vi "CIETallnodesReactor.vi"() -> ()   [LabVIEW 2017]
uses:
  <vilib>/OPCUA/controls/Write Status.ctl
  <vilib>/OPCUA/controls/NodeId.ctl
  <vilib>/OPCUA/controls/Subscription Data Change.ctl
  <vilib>/OPCUA/controls/Data Type.ctl
  <vilib>/OPCUA/controls/OPC UA StatusCode.ctl
  <vilib>/OPCUA/controls/Subscription ID.ctl
  <vilib>/OPCUA/controls/OPC UA Client Refnum.ctl
  <vilib>/OPCUA/controls/NodeIds.ctl
  <vilib>/OPCUA/client/Multiple Write Bool.vi
  <vilib>/OPCUA/client/Multiple Write Double.vi
  <vilib>/OPCUA/NI OPC UA Client.lvlib
panel:
  out "CX-114":dbl format="%.1f"
  out "CX-113":dbl format="%.1f"
  out "CX-112":dbl format="%.1f"
  out "CX-111":dbl format="%.1f"
  out "CX-104":dbl format="%.1f"
  out "CX-103":dbl format="%.1f"
  out "CX-102":dbl format="%.1f"
  out "CX-101":dbl format="%.1f"
  out "ST-14w":dbl format="%.1f"
  out "ST-14s":dbl format="%.1f"
  out "ST-14n":dbl format="%.1f"
  out "ST-14e":dbl format="%.1f"
  out "ST-12sw":dbl format="%.1f"
  out "ST-12se":dbl format="%.1f"
  out "ST-12n":dbl format="%.1f"
  in  "Flow Data?":bool=TRUE
  in  "CTAH Set Point":sgl format="%.1f"
  in  "Mode":string(combo)
  out "Server OK":bool
  out "System Time [s]":dbl
  out "Power Output":dbl(graph)
  out "Frequency [Hz] 3":dbl(slide) scale=0.0..60.0
  out "Frequency [Hz] 2":dbl(slide) scale=0.0..60.0
  out "Frequency [Hz]":dbl(knob) scale=0.0..45.0
  out "Power [W]":dbl(slide) caption="Power Output [W]" scale=0.0..10000.0
  in  "Desired Power [W]":dbl min=0.0 max=10000.0 step=1.0 format="%.1f"
  out "WT-10":dbl format="%.1f"
  out "BT-11":dbl format="%.1f"
  out "BT-12":dbl format="%.1f"
  out "WT-13":dbl format="%.1f"
  out "WT-20":dbl format="%.1f"
  out "BT-21":dbl format="%.1f"
  out "WT-22":dbl format="%.1f"
  out "BT-23":dbl format="%.1f"
  out "WT-24":dbl format="%.1f"
  out "BT-25":dbl format="%.1f"
  out "WT-26":dbl format="%.1f"
  out "BT-27":dbl format="%.1f"
  out "WT-28":dbl format="%.1f"
  out "BT-29":sgl format="%.1f"
  out "BT-30":dbl format="%.1f"
  out "WT-31":dbl format="%.1f"
  out "BT-32":dbl format="%.1f"
  out "WT-33":dbl format="%.1f"
  out "BT-34":dbl format="%.1f"
  out "WT-35":dbl format="%.1f"
  out "WT-40":dbl format="%.1f"
  out "BT-41":dbl format="%.1f"
  out "WT-42":dbl format="%.1f"
  out "BT-43":dbl format="%.1f"
  out "BT-60":dbl format="%.1f"
  out "WT-61":dbl format="%.1f"
  out "WT-62":dbl format="%.1f"
  out "BT-63":dbl format="%.1f"
  out "WT-64":dbl format="%.1f"
  out "BT-65":sgl format="%.1f"
  out "BT-66":dbl format="%.1f"
  out "WT-67":dbl format="%.1f"
  out "ST-10":dbl format="%.1f"
  out "ST-11":dbl format="%.1f"
  out "ST-13":dbl format="%.1f"
  out "AT-01":dbl format="%.1f"
  out "AT-02":dbl format="%.1f"
  in  "Power Output On":bool
  in  "ACTIVATE - CTAH":bool
  in  "ACTIVATE - TCHX":bool
  in  "TCHX Frequency [Hz]":sgl min=0 max=60 step=0.1 format="%.1f"
  in  "ACTIVATE - PUMP":bool
  in  "Pump Frequency [Hz]":dbl min=0.0 max=45.0 step=0.10000000149011612 format="%.1f"
  out "DHX Primary Flow\n\n\nFM-20 [kg/s]":dbl format="%.3f"
  out "Bypass Flow\n\n\nFM-30 [kg/s]":dbl format="%.3f"
  out "Primary Flow\n\n\nFM-40 [kg/s]":dbl format="%.3f"
  out "DRACS Flow\n\n\nFM-60 [kg/s]":dbl format="%.3f"
  out "System Safe":bool
  in  "Exit Profile":bool
  in  "Select Operation Mode":T1(ring) caption="Select Operation Mode2"
  in  "Load Power Profile":bool
  in  "Dyn. Power Profile File":path
  out "CTAH Temperatures":cluster{"CTAH Outlet":dbl, "CTAH Inlet":dbl}(graph)
  out "Core Temperatures":cluster{"Heater Inlet":dbl, "Heater Outlet":dbl}(graph)
  out "Profile Step":i32
  in  "Stop Reactor Interface":bool
  in  "error in (no error)":errorcluster
  out "Connection Status":bool
  in  "Stop":bool
  in  "Disconnect":bool
  in  "Connect to Server":bool
  out "activateTchx":bool
  out "activatePump":bool
  out "activateCtah":bool
  out "20001":dbl
  out "operatorActions":string
  out "chat":string
  out "spoofEnabled":bool
  out "flowData":dbl
  out "exitProfile":bool
  out "actionRecorderOn":bool
  out "powerOutputOn":bool
  out "powerInputSignal":dbl
  out "outputVoltage2":dbl
  out "outputVoltage1":dbl
  out "outputCurrent2":dbl
  out "outputCurrent1":dbl
  out "tchxTempInResGen":dbl
  out "matlabActive":bool
  out "heaterTempOutResGen":dbl
  out "heaterResGen":dbl
  out "faultDiagnosticsActive":bool
  out "dhxTempOutResGen":dbl
  out "ctahTempInResGen":dbl
  out "CTAHResGen":bool
  out "Temperature":dbl
  out "Message":string
  out "Sensor Status":bool
  out "Time Stamp 2":timestamp
  # "DRACS"
  # "PRIMARY"
  # "HOT DRACS"
  # "DHX TOP"
  # "TCHX"
  # "HOT LEG"
  # "COLD DRACS"
  # "DHX"
  # "BYPASS"
  # "CTAH"
  # "HEATER"
  # "DHX BOTTOM"
  # "COLD LEG"
  # "PUMP"
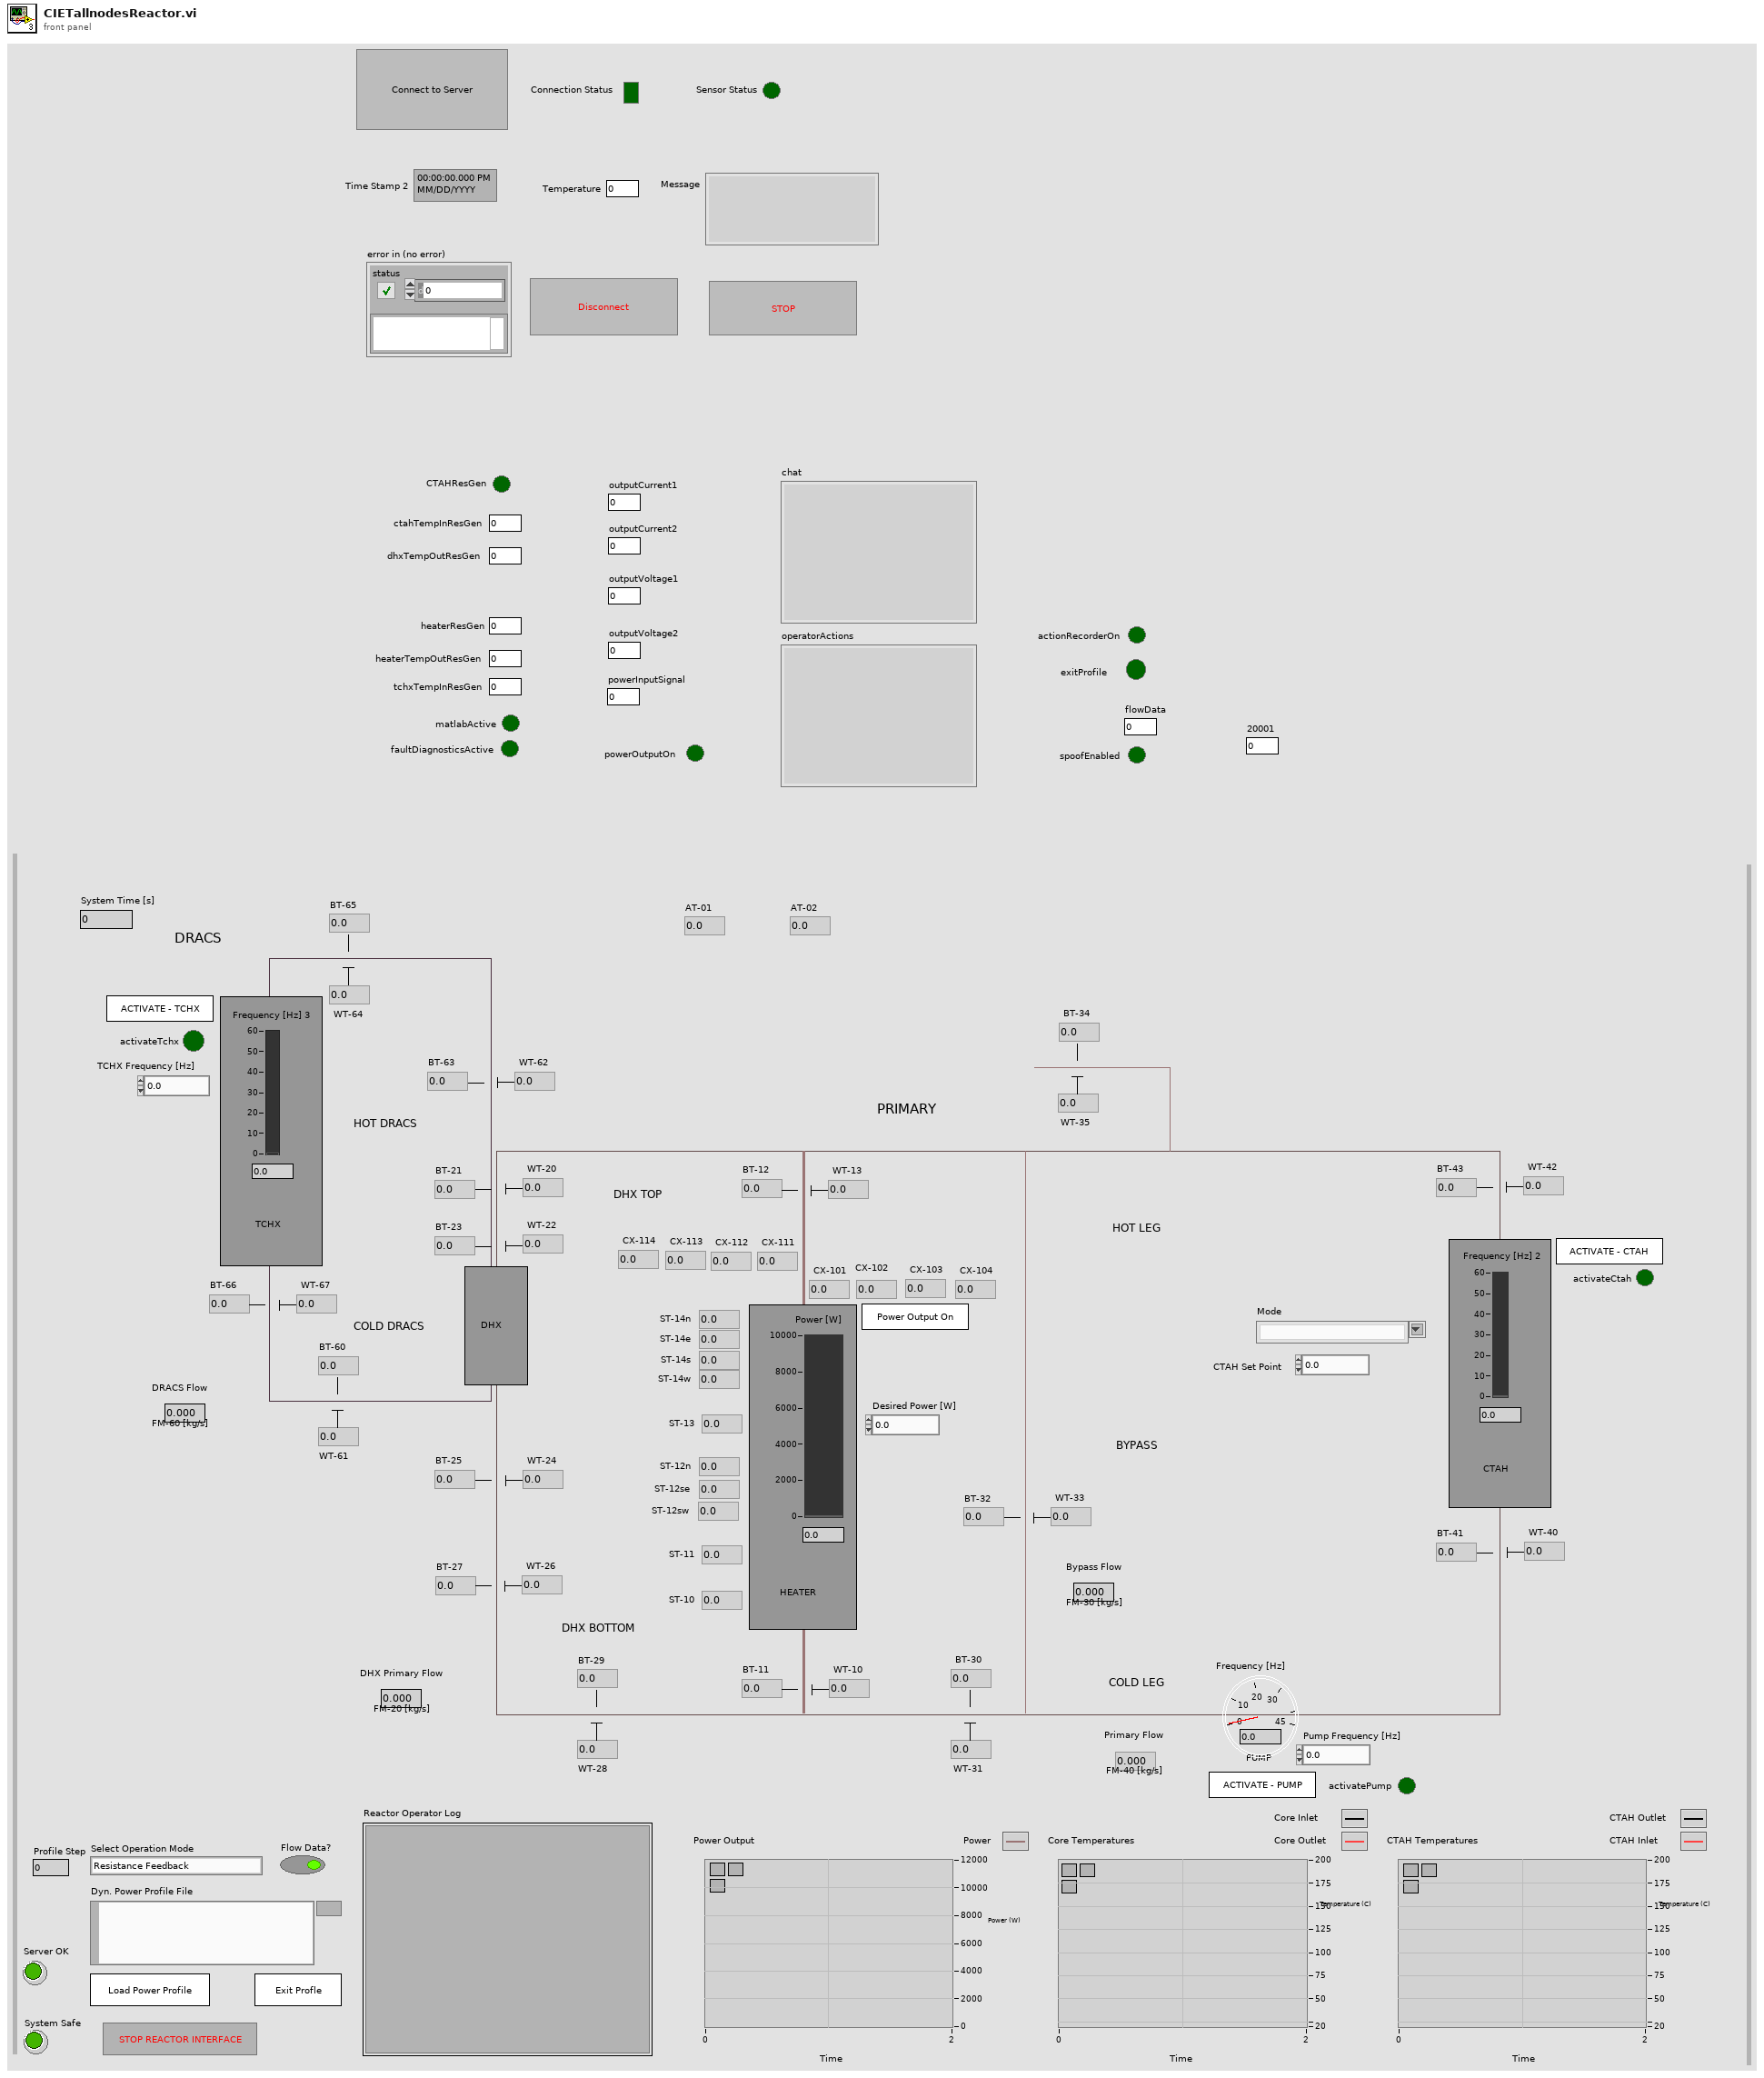
[diagram p1: front panel]
types:
  T1 = enum16{"Resistance Feedback", "Power Profile Input", "Resistance Feedback_Analog", "Power Profile Input_Analog", "Shutdown"}
  T2 = typedef "NodeId.ctl" = string
  T3 = typedef "Write Status.ctl" = u32
  T4 = cluster{"node ID":T2, "value":bool, "timestamp (current time)":timestamp, "node status":T3}
  T5 = cluster{"node ID":T2, "value":dbl, "timestamp (current time)":timestamp, "node status":T3}
  T6 = cluster{"message mode":enum16{"None", "Sign", "Sign and Encrypt"}, "security":enum16{"Basic256", "Basic128Rsa15"}}
  T7 = typedef "OPC UA Client Refnum.ctl" = refnum<k21>
  T8 = typedef "Subscription Data Change.ctl" = cluster{"node ID":T2, " value":variant, "timestamp":timestamp, "data type":T9, "status code":T10}
  T9 = typedef "Data Type.ctl" = u16
  T10 = typedef "OPC UA StatusCode.ctl" = u32
  T11 = cluster{"node ID":T2, "value":bool, "timestamp (current time)":timestamp, "node status":T3}[]
  T12 = cluster{"node ID":T2, "value":dbl, "timestamp (current time)":timestamp, "node status":T3}[]
  T13 = typedef "Subscription ID.ctl" = u32
  T14 = cluster{"OPC UA Data Change Event Registration Refnum":refnum<event-registration>, "OPC UA client refnum ":T7, "OPC UA Subscription Service Status":T10, "OPC UA Subscription ID":T13, "OPC UA Monitored Nodes":string[], "Connection Status":bool}
  T15 = typedef "NodeIds.ctl" = T2[]
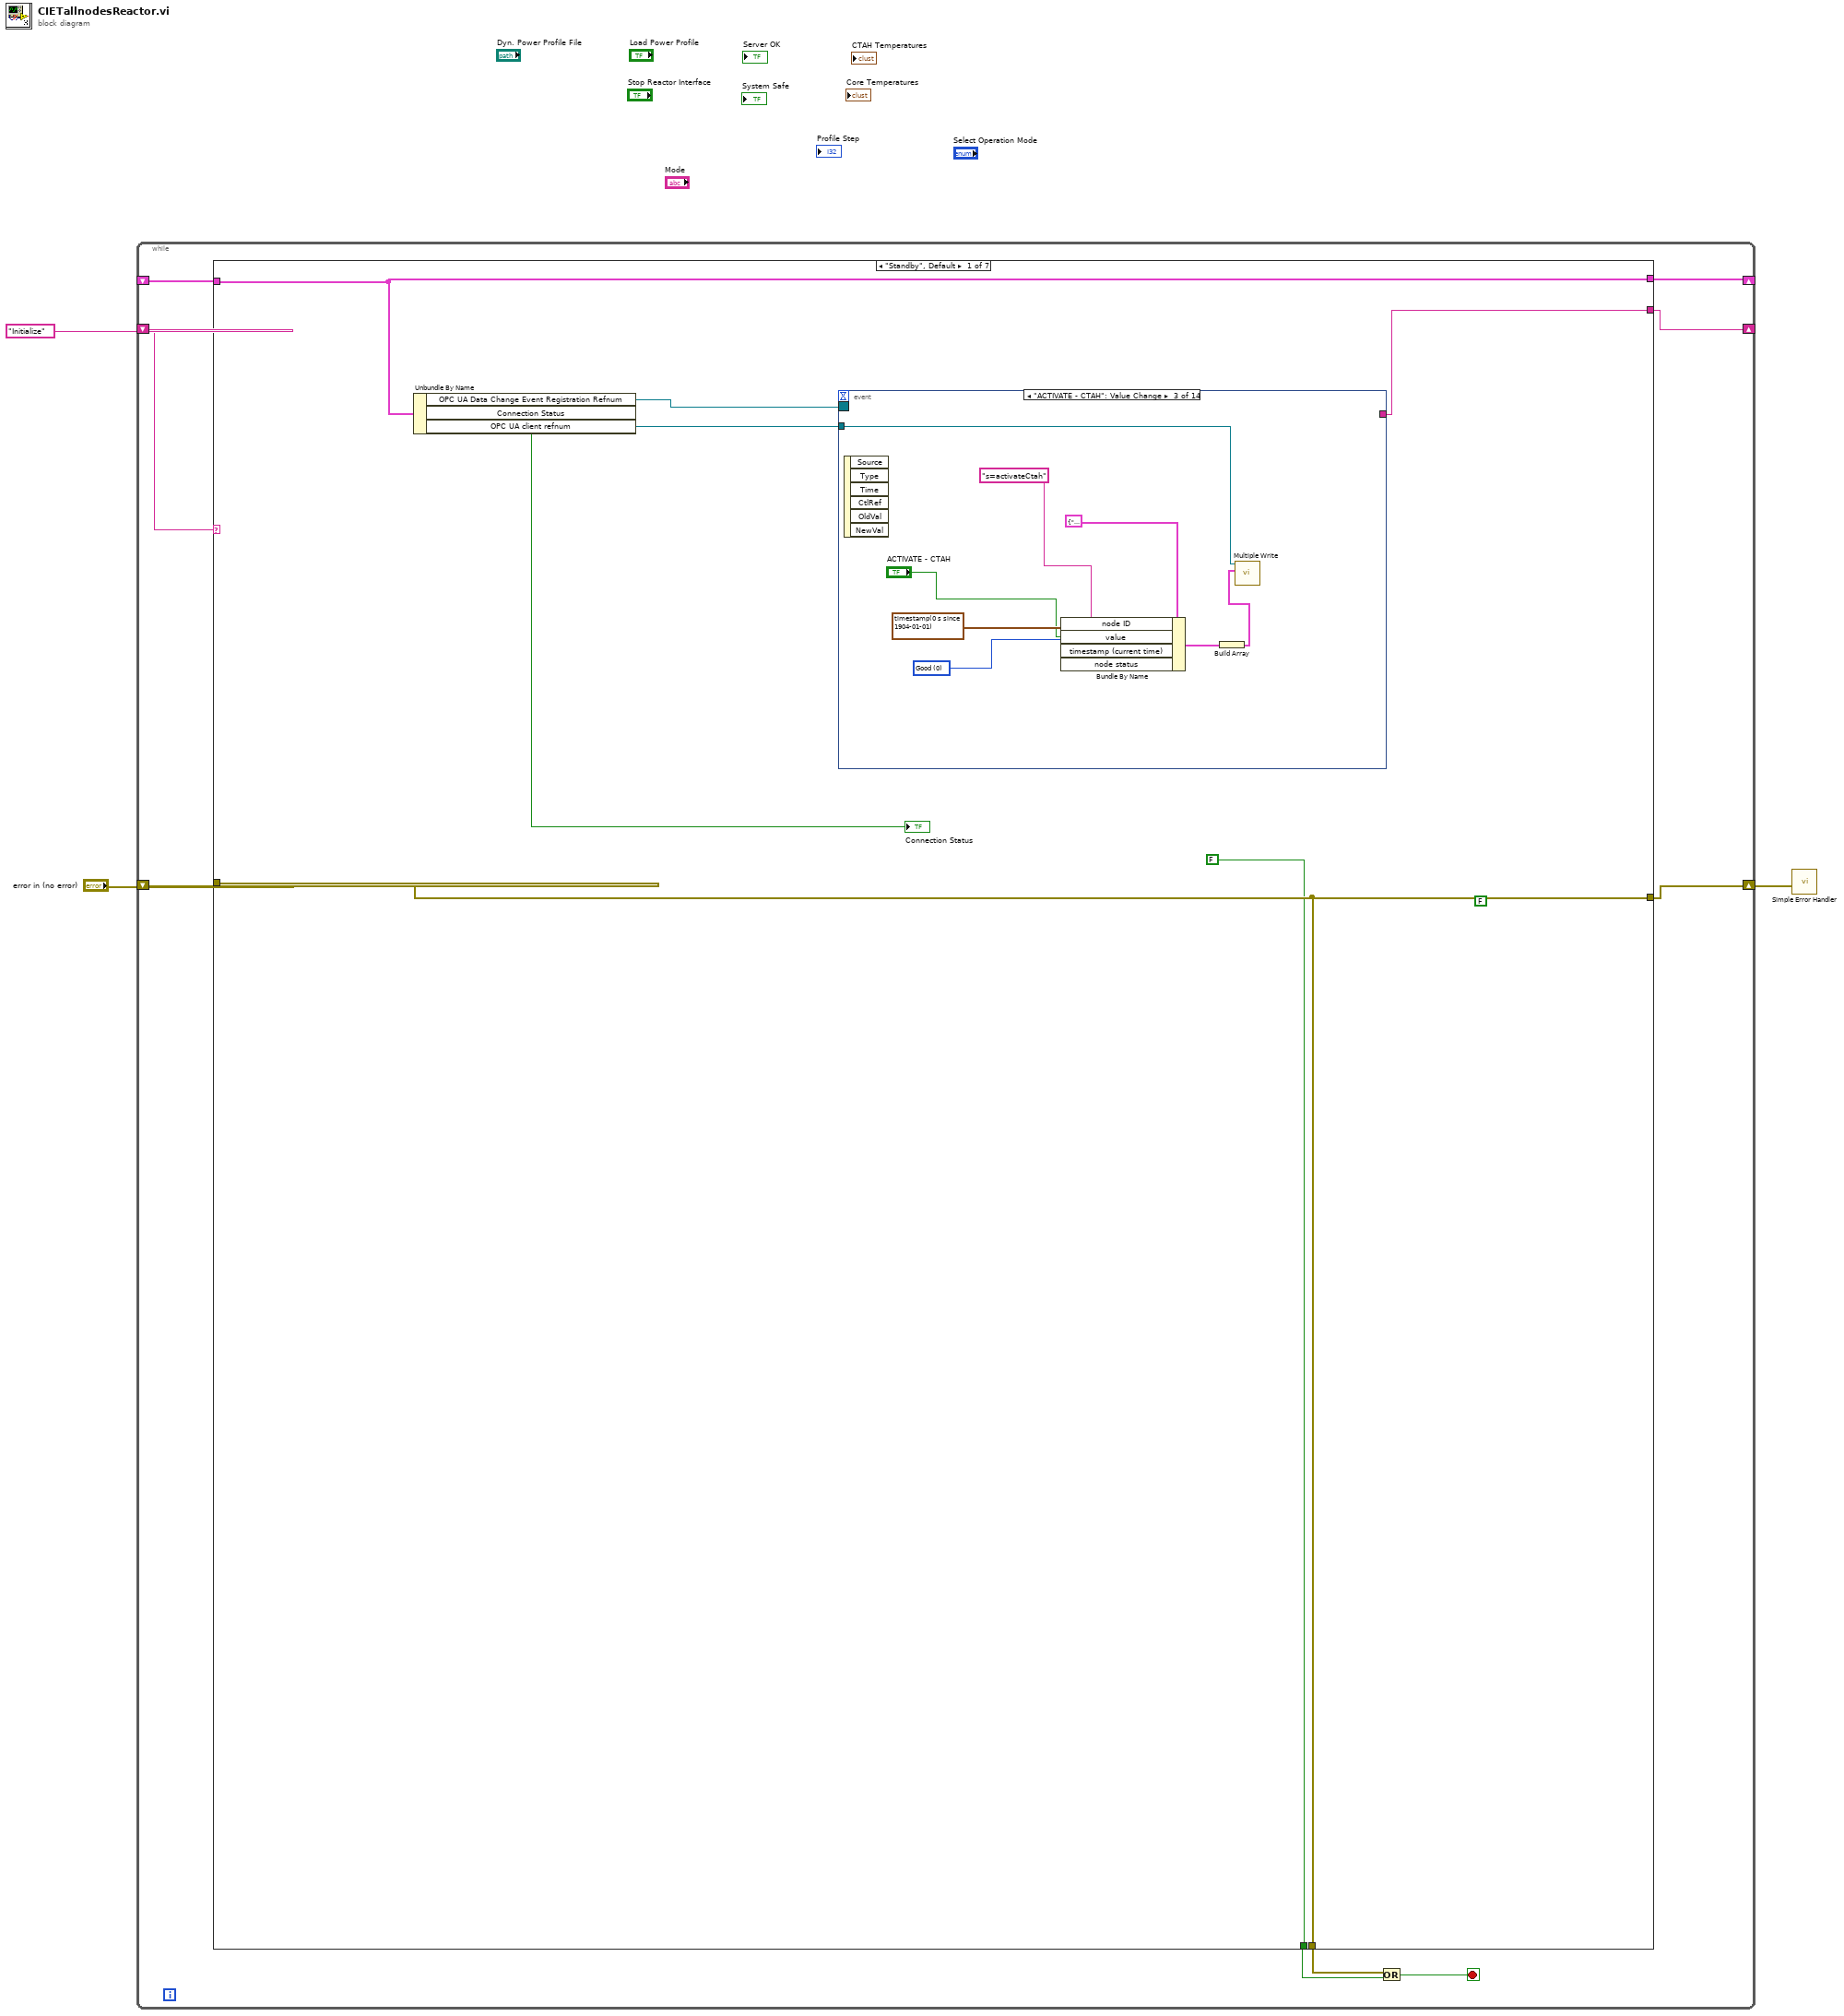
[diagram p0: block diagram]
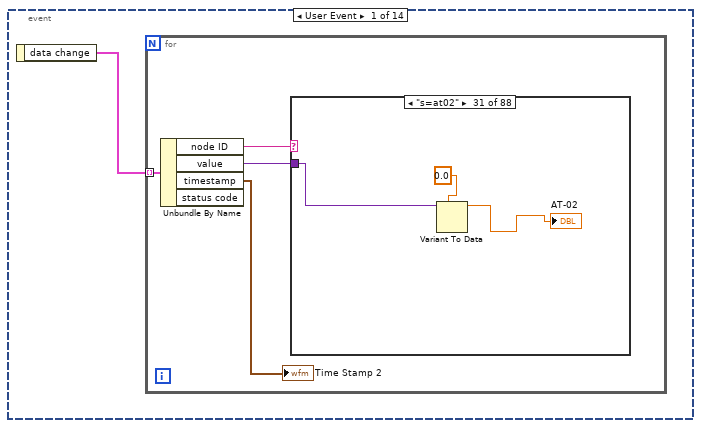
[diagram p2: hidden frame]
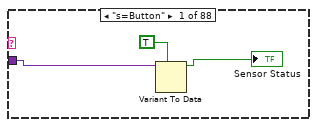
[diagram p3: hidden frame]
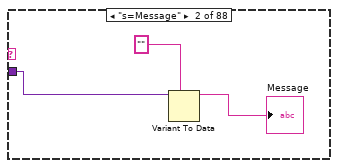
[diagram p4: hidden frame]
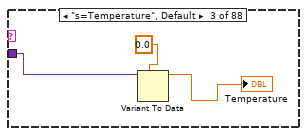
[diagram p5: hidden frame]
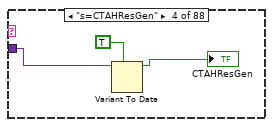
[diagram p6: hidden frame]
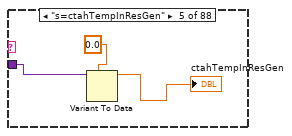
[diagram p7: hidden frame]
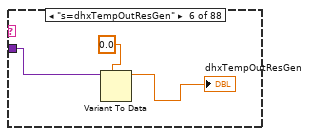
[diagram p8: hidden frame]
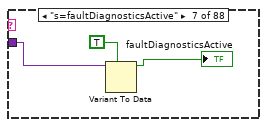
[diagram p9: hidden frame]
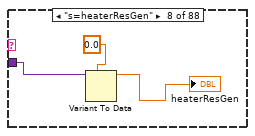
[diagram p10: hidden frame]
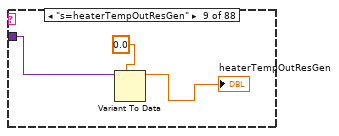
[diagram p11: hidden frame]
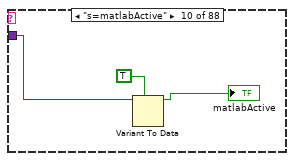
[diagram p12: hidden frame]
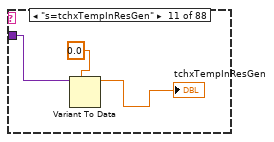
[diagram p13: hidden frame]
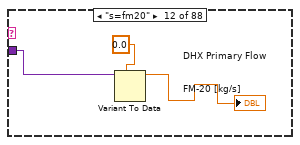
[diagram p14: hidden frame]
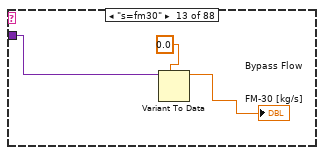
[diagram p15: hidden frame]
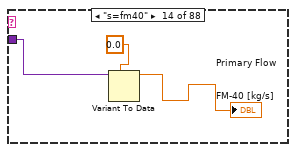
[diagram p16: hidden frame]
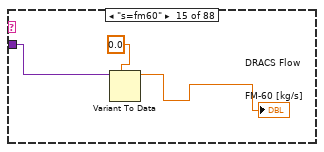
[diagram p17: hidden frame]
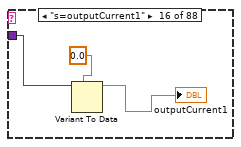
[diagram p18: hidden frame]
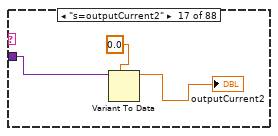
[diagram p19: hidden frame]
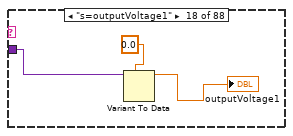
[diagram p20: hidden frame]
diagram:
  n1 = while {
    shift-right: [w7] -> _
    shift-left: _ -> [w8]
    shift-right: [w6] -> w2
    shift-left: "error in (no error)" -> [w12]
    shift-right: [w4] -> _
    shift-left: "Initialize" -> [w5]
    stop <- w10 stop-if-true
    n2 = case shown="\"Standby\", Default" w5 {
      tunnel: w12 -> [w15 w373 w391 w405 w424 w439 w448]
      tunnel: [w15 w373 w385 w405 w419 w434 w448] -> w11
      tunnel: [FALSE FALSE FALSE FALSE FALSE FALSE TRUE] -> w9
      tunnel: [w17 "Standby" "Standby" w406 "Standby" "Stop" "Initialize"] -> w4
      tunnel: [w16 w375 w384 w404 w417 w432 w447] -> w7
      tunnel: w8 -> [w16 w374 w387 w404 w418 w433 w447]
      tunnel: [w15 w373 w385 w405 w419 w434 w448] -> w6
      frame "Standby", Default {
        (unwired) FALSE
        n3 = Unbundle By Name(w16) -> ("OPC UA Data Change Event Registration Refnum"=w18:refnum<event-registration>, "Connection Status"=→"Connection Status":bool, "OPC UA client refnum"=w13:T7)
        n4 = event shown="[2] \"ACTIVATE - CTAH\": Value Change" {
          selector: w18 -> [_ _ _ _ _ _ _ _ _ _ _ _ _ _]
          dyn-events: _ -> [_ _ _ _ _ _ _ _ _ _ _ _ _ _]
          timeout: _ -> [_ _ _ _ _ _ _ _ _ _ _ _ _ _]
          tunnel: [_ _ _ _ _ _ _ _ _ _ _ "Connect" "Disconnect" "Stop Check"] -> w17
          tunnel: w13 -> [_ w296 w297 w305 w317 w321 w329 w337 w345 w353 w361 _ _ _]
          event User Event {
            n5 = event-data() -> ("data change"=w20:T8[])  [unwired: 1 in]
            n6 = for {
              tunnel: w20 -> [w23] mode=indexing
              n7 = Unbundle By Name(w23) -> ("node ID"=w22:T2, "value"=w21:variant, "timestamp"=→"Time Stamp 2":timestamp)  [unwired: 1 out]
              n8 = case shown="\"s=at02\"" w22 {
                tunnel: w21 -> [w25 w28 w31 w34 w37 w40 w43 w46 w49 w52 w55 w59 w62 w65 w68 w70 w73 w76 w79 w82 w86 w88 w91 w94 w97 w100 w104 w106 w109 w113 w115 w118 w122 w125 w128 w131 w134 w137 w140 w143 w146 w149 w152 w155 w158 w161 w164 w167 w170 w173 w176 w179 w182 w185 w188 w191 w194 w197 w200 w203 w206 w209 w212 w215 w218 w221 w224 w227 w230 w233 w236 w239 w242 w245 w248 w251 w254 w257 w260 w263 w266 w269 w273 w274 w277 w281 w284 w287]
                frame "s=Button" {
                  n9 = Variant To Data(type=TRUE, Variant=w25) -> (data=→"Sensor Status":bool)  [unwired: 1 in, 1 out]
                }
                frame "s=Message" {
                  n10 = Variant To Data(type="", Variant=w28) -> (data=→"Message":string)  [unwired: 1 in, 1 out]
                }
                frame "s=Temperature", Default {
                  n11 = Variant To Data(type=0.0, Variant=w31) -> (data=→"Temperature":dbl)  [unwired: 1 in, 1 out]
                }
                frame "s=CTAHResGen" {
                  n12 = Variant To Data(type=TRUE, Variant=w34) -> (data=→"CTAHResGen":bool)  [unwired: 1 in, 1 out]
                }
                frame "s=ctahTempInResGen" {
                  n13 = Variant To Data(type=0.0, Variant=w37) -> (data=→"ctahTempInResGen":dbl)  [unwired: 1 in, 1 out]
                }
                frame "s=dhxTempOutResGen" {
                  n14 = Variant To Data(type=0.0, Variant=w40) -> (data=→"dhxTempOutResGen":dbl)  [unwired: 1 in, 1 out]
                }
                frame "s=faultDiagnosticsActive" {
                  n15 = Variant To Data(type=TRUE, Variant=w43) -> (data=→"faultDiagnosticsActive":bool)  [unwired: 1 in, 1 out]
                }
                frame "s=heaterResGen" {
                  n16 = Variant To Data(type=0.0, Variant=w46) -> (data=→"heaterResGen":dbl)  [unwired: 1 in, 1 out]
                }
                frame "s=heaterTempOutResGen" {
                  n17 = Variant To Data(type=0.0, Variant=w49) -> (data=→"heaterTempOutResGen":dbl)  [unwired: 1 in, 1 out]
                }
                frame "s=matlabActive" {
                  n18 = Variant To Data(type=TRUE, Variant=w52) -> (data=→"matlabActive":bool)  [unwired: 1 in, 1 out]
                }
                frame "s=tchxTempInResGen" {
                  n19 = Variant To Data(type=0.0, Variant=w55) -> (data=→"tchxTempInResGen":dbl)  [unwired: 1 in, 1 out]
                }
                frame "s=fm20" {
                  n20 = Variant To Data(type=0.0, Variant=w59) -> (data=→"DHX Primary Flow\n\n\nFM-20 [kg/s]":dbl)  [unwired: 1 in, 1 out]
                }
                frame "s=fm30" {
                  n21 = Variant To Data(type=0.0, Variant=w62) -> (data=→"Bypass Flow\n\n\nFM-30 [kg/s]":dbl)  [unwired: 1 in, 1 out]
                }
                frame "s=fm40" {
                  n22 = Variant To Data(type=0.0, Variant=w65) -> (data=→"Primary Flow\n\n\nFM-40 [kg/s]":dbl)  [unwired: 1 in, 1 out]
                }
                frame "s=fm60" {
                  n23 = Variant To Data(type=0.0, Variant=w68) -> (data=→"DRACS Flow\n\n\nFM-60 [kg/s]":dbl)  [unwired: 1 in, 1 out]
                }
                frame "s=outputCurrent1" {
                  n24 = Variant To Data(type=0.0, Variant=w70) -> (data=→"outputCurrent1":dbl)  [unwired: 1 in, 1 out]
                }
                frame "s=outputCurrent2" {
                  n25 = Variant To Data(type=0.0, Variant=w73) -> (data=→"outputCurrent2":dbl)  [unwired: 1 in, 1 out]
                }
                frame "s=outputVoltage1" {
                  n26 = Variant To Data(type=0.0, Variant=w76) -> (data=→"outputVoltage1":dbl)  [unwired: 1 in, 1 out]
                }
                frame "s=outputVoltage2" {
                  n27 = Variant To Data(type=0.0, Variant=w79) -> (data=→"outputVoltage2":dbl)  [unwired: 1 in, 1 out]
                }
                frame "s=powerInputSignal" {
                  n28 = Variant To Data(type=0.0, Variant=w82) -> (data=→"powerInputSignal":dbl)  [unwired: 1 in, 1 out]
                }
                frame "s=powerOutput" {
                  n29 = Variant To Data(type=0.0, Variant=w86) -> (data=→"Power [W]" →"Power Output":dbl)  [unwired: 1 in, 1 out]
                }
                frame "s=powerOutputOn" {
                  n30 = Variant To Data(type=TRUE, Variant=w88) -> (data=→"powerOutputOn":bool)  [unwired: 1 in, 1 out]
                }
                frame "s=actionRecorderOn" {
                  n31 = Variant To Data(type=TRUE, Variant=w91) -> (data=→"actionRecorderOn":bool)  [unwired: 1 in, 1 out]
                }
                frame "s=exitProfile" {
                  n32 = Variant To Data(type=TRUE, Variant=w94) -> (data=→"exitProfile":bool)  [unwired: 1 in, 1 out]
                }
                frame "s=flowData" {
                  n33 = Variant To Data(type=0.0, Variant=w97) -> (data=→"flowData":dbl)  [unwired: 1 in, 1 out]
                }
                frame "s=spoofEnabled" {
                  n34 = Variant To Data(type=TRUE, Variant=w100) -> (data=→"spoofEnabled":bool)  [unwired: 1 in, 1 out]
                }
                frame "s=time" {
                  n35 = Variant To Data(type=0.0, Variant=w104) -> (data=→"System Time [s]":dbl)  [unwired: 1 in, 1 out]
                }
                frame "s=chat" {
                  n36 = Variant To Data(type="", Variant=w106) -> (data=→"chat":string)  [unwired: 1 in, 1 out]
                }
                frame "s=operatorActions" {
                  n37 = Variant To Data(type="", Variant=w109) -> (data=→"operatorActions":string)  [unwired: 1 in, 1 out]
                }
                frame "s=at01" {
                  n38 = Variant To Data(type=0.0, Variant=w113) -> (data=→"AT-01":dbl)  [unwired: 1 in, 1 out]
                }
                frame "s=at02" {
                  n39 = Variant To Data(type=0.0, Variant=w115) -> (data=→"AT-02":dbl)  [unwired: 1 in, 1 out]
                }
                frame "i=20001" {
                  n40 = Variant To Data(type=0.0, Variant=w118) -> (data=→"20001":dbl)  [unwired: 1 in, 1 out]
                }
                frame "s=bt11" {
                  n41 = Variant To Data(type=0.0, Variant=w122) -> (data=→"BT-11":dbl)  [unwired: 1 in, 1 out]
                }
                frame "s=bt12" {
                  n42 = Variant To Data(type=0.0, Variant=w125) -> (data=→"BT-12":dbl)  [unwired: 1 in, 1 out]
                }
                frame "s=bt21" {
                  n43 = Variant To Data(type=0.0, Variant=w128) -> (data=→"BT-21":dbl)  [unwired: 1 in, 1 out]
                }
                frame "s=bt23" {
                  n44 = Variant To Data(type=0.0, Variant=w131) -> (data=→"BT-23":dbl)  [unwired: 1 in, 1 out]
                }
                frame "s=bt25" {
                  n45 = Variant To Data(type=0.0, Variant=w134) -> (data=→"BT-25":dbl)  [unwired: 1 in, 1 out]
                }
                frame "s=bt27" {
                  n46 = Variant To Data(type=0.0, Variant=w137) -> (data=→"BT-27":dbl)  [unwired: 1 in, 1 out]
                }
                frame "s=bt29" {
                  n47 = Variant To Data(type=0.0, Variant=w140) -> (data=→"BT-29":dbl)  [unwired: 1 in, 1 out]
                }
                frame "s=bt30" {
                  n48 = Variant To Data(type=0.0, Variant=w143) -> (data=→"BT-30":dbl)  [unwired: 1 in, 1 out]
                }
                frame "s=bt32" {
                  n49 = Variant To Data(type=0.0, Variant=w146) -> (data=→"BT-32":dbl)  [unwired: 1 in, 1 out]
                }
                frame "s=bt34" {
                  n50 = Variant To Data(type=0.0, Variant=w149) -> (data=→"BT-34":dbl)  [unwired: 1 in, 1 out]
                }
                frame "s=bt41" {
                  n51 = Variant To Data(type=0.0, Variant=w152) -> (data=→"BT-41":dbl)  [unwired: 1 in, 1 out]
                }
                frame "s=bt43" {
                  n52 = Variant To Data(type=0.0, Variant=w155) -> (data=→"BT-43":dbl)  [unwired: 1 in, 1 out]
                }
                frame "s=bt60" {
                  n53 = Variant To Data(type=0.0, Variant=w158) -> (data=→"BT-60":dbl)  [unwired: 1 in, 1 out]
                }
                frame "s=bt63" {
                  n54 = Variant To Data(type=0.0, Variant=w161) -> (data=→"BT-63":dbl)  [unwired: 1 in, 1 out]
                }
                frame "s=bt65" {
                  n55 = Variant To Data(type=0.0, Variant=w164) -> (data=→"BT-65":dbl)  [unwired: 1 in, 1 out]
                }
                frame "s=bt66" {
                  n56 = Variant To Data(type=0.0, Variant=w167) -> (data=→"BT-66":dbl)  [unwired: 1 in, 1 out]
                }
                frame "s=cx101" {
                  n57 = Variant To Data(type=0.0, Variant=w170) -> (data=→"CX-101":dbl)  [unwired: 1 in, 1 out]
                }
                frame "s=cx102" {
                  n58 = Variant To Data(type=0.0, Variant=w173) -> (data=→"CX-102":dbl)  [unwired: 1 in, 1 out]
                }
                frame "s=cx103" {
                  n59 = Variant To Data(type=0.0, Variant=w176) -> (data=→"CX-103":dbl)  [unwired: 1 in, 1 out]
                }
                frame "s=cx104" {
                  n60 = Variant To Data(type=0.0, Variant=w179) -> (data=→"CX-104":dbl)  [unwired: 1 in, 1 out]
                }
                frame "s=cx111" {
                  n61 = Variant To Data(type=0.0, Variant=w182) -> (data=→"CX-111":dbl)  [unwired: 1 in, 1 out]
                }
                frame "s=cx112" {
                  n62 = Variant To Data(type=0.0, Variant=w185) -> (data=→"CX-112":dbl)  [unwired: 1 in, 1 out]
                }
                frame "s=cx113" {
                  n63 = Variant To Data(type=0.0, Variant=w188) -> (data=→"CX-113":dbl)  [unwired: 1 in, 1 out]
                }
                frame "s=cx114" {
                  n64 = Variant To Data(type=0.0, Variant=w191) -> (data=→"CX-114":dbl)  [unwired: 1 in, 1 out]
                }
                frame "s=st10" {
                  n65 = Variant To Data(type=0.0, Variant=w194) -> (data=→"ST-10":dbl)  [unwired: 1 in, 1 out]
                }
                frame "s=st11" {
                  n66 = Variant To Data(type=0.0, Variant=w197) -> (data=→"ST-11":dbl)  [unwired: 1 in, 1 out]
                }
                frame "s=st12n" {
                  n67 = Variant To Data(type=0.0, Variant=w200) -> (data=→"ST-12n":dbl)  [unwired: 1 in, 1 out]
                }
                frame "s=st12se" {
                  n68 = Variant To Data(type=0.0, Variant=w203) -> (data=→"ST-12se":dbl)  [unwired: 1 in, 1 out]
                }
                frame "s=st12sw" {
                  n69 = Variant To Data(type=0.0, Variant=w206) -> (data=→"ST-12sw":dbl)  [unwired: 1 in, 1 out]
                }
                frame "s=st13" {
                  n70 = Variant To Data(type=0.0, Variant=w209) -> (data=→"ST-13":dbl)  [unwired: 1 in, 1 out]
                }
                frame "s=st14e" {
                  n71 = Variant To Data(type=0.0, Variant=w212) -> (data=→"ST-14e":dbl)  [unwired: 1 in, 1 out]
                }
                frame "s=st14n" {
                  n72 = Variant To Data(type=0.0, Variant=w215) -> (data=→"ST-14n":dbl)  [unwired: 1 in, 1 out]
                }
                frame "s=st14s" {
                  n73 = Variant To Data(type=0.0, Variant=w218) -> (data=→"ST-14s":dbl)  [unwired: 1 in, 1 out]
                }
                frame "s=st14w" {
                  n74 = Variant To Data(type=0.0, Variant=w221) -> (data=→"ST-14w":dbl)  [unwired: 1 in, 1 out]
                }
                frame "s=wt10" {
                  n75 = Variant To Data(type=0.0, Variant=w224) -> (data=→"WT-10":dbl)  [unwired: 1 in, 1 out]
                }
                frame "s=wt13" {
                  n76 = Variant To Data(type=0.0, Variant=w227) -> (data=→"WT-13":dbl)  [unwired: 1 in, 1 out]
                }
                frame "s=wt20" {
                  n77 = Variant To Data(type=0.0, Variant=w230) -> (data=→"WT-20":dbl)  [unwired: 1 in, 1 out]
                }
                frame "s=wt22" {
                  n78 = Variant To Data(type=0.0, Variant=w233) -> (data=→"WT-22":dbl)  [unwired: 1 in, 1 out]
                }
                frame "s=wt24" {
                  n79 = Variant To Data(type=0.0, Variant=w236) -> (data=→"WT-24":dbl)  [unwired: 1 in, 1 out]
                }
                frame "s=wt26" {
                  n80 = Variant To Data(type=0.0, Variant=w239) -> (data=→"WT-26":dbl)  [unwired: 1 in, 1 out]
                }
                frame "s=wt28" {
                  n81 = Variant To Data(type=0.0, Variant=w242) -> (data=→"WT-28":dbl)  [unwired: 1 in, 1 out]
                }
                frame "s=wt31" {
                  n82 = Variant To Data(type=0.0, Variant=w245) -> (data=→"WT-31":dbl)  [unwired: 1 in, 1 out]
                }
                frame "s=wt33" {
                  n83 = Variant To Data(type=0.0, Variant=w248) -> (data=→"WT-33":dbl)  [unwired: 1 in, 1 out]
                }
                frame "s=wt35" {
                  n84 = Variant To Data(type=0.0, Variant=w251) -> (data=→"WT-35":dbl)  [unwired: 1 in, 1 out]
                }
                frame "s=wt40" {
                  n85 = Variant To Data(type=0.0, Variant=w254) -> (data=→"WT-40":dbl)  [unwired: 1 in, 1 out]
                }
                frame "s=wt42" {
                  n86 = Variant To Data(type=0.0, Variant=w257) -> (data=→"WT-42":dbl)  [unwired: 1 in, 1 out]
                }
                frame "s=wt61" {
                  n87 = Variant To Data(type=0.0, Variant=w260) -> (data=→"WT-61":dbl)  [unwired: 1 in, 1 out]
                }
                frame "s=wt62" {
                  n88 = Variant To Data(type=0.0, Variant=w263) -> (data=→"WT-62":dbl)  [unwired: 1 in, 1 out]
                }
                frame "s=wt64" {
                  n89 = Variant To Data(type=0.0, Variant=w266) -> (data=→"WT-64":dbl)  [unwired: 1 in, 1 out]
                }
                frame "s=wt67" {
                  n90 = Variant To Data(type=0.0, Variant=w269) -> (data=→"WT-67":dbl)  [unwired: 1 in, 1 out]
                }
                frame "s=activateCtah" {
                  n91 = Variant To Data(type=TRUE, Variant=w273) -> (data=→"activateCtah":bool)  [unwired: 1 in, 1 out]
                }
                frame "s=activatePump" {
                  n92 = Variant To Data(type=TRUE, Variant=w274) -> (data=→"activatePump":bool)  [unwired: 1 in, 1 out]
                }
                frame "s=activateTchx" {
                  n93 = Variant To Data(type=TRUE, Variant=w277) -> (data=→"activateTchx":bool)  [unwired: 1 in, 1 out]
                }
                frame "s=ctahFrequency" {
                  n94 = Variant To Data(type=0.0, Variant=w281) -> (data=→"Frequency [Hz] 2":dbl)  [unwired: 1 in, 1 out]
                }
                frame "s=pumpFrequency" {
                  n95 = Variant To Data(type=0.0, Variant=w284) -> (data=→"Frequency [Hz]":dbl)  [unwired: 1 in, 1 out]
                }
                frame "s=tchxFrequency" {
                  n96 = Variant To Data(type=0.0, Variant=w287) -> (data=→"Frequency [Hz] 3":dbl)  [unwired: 1 in, 1 out]
                }
              }
            }
          }
          event "ACTIVATE - TCHX": Value Change {
            w293 = T3 0 items=["Good"=0, "Uncertain_InitialValue"=1083310080, "Uncertain_LastUsableValue"=1083179008, "Uncertain_SensorNotAccurate"=1083375616, "Uncertain_EngineeringUnitsExceeded"=1083441152, "Bad_NoCommunication"=2150694912, "Bad_NotReadable"=2151284736, "Bad_NotWritable"=2151350272, "Bad_OutOfRange"=2151415808, "Bad_WaitingForInitialData"=2150760448] ("node status")
            n97 = event-data() -> ()  [unwired: 1 in, 6 out]
            n98 = Bundle By Name(cluster=T4 {"node ID"="", "value"=FALSE, "timestamp (current time)"=timestamp(0 s since 1904-01-01), "node status"=0} ("request"), "node ID"="s=activateTchx", "value"="ACTIVATE - TCHX", "timestamp (current time)"=timestamp(0 s since 1904-01-01), "node status"=w293) -> (w290:T4)
            n99 = Build Array(w290) -> (w289:T11)
            n100 = call-poly <vilib>:"Multiple Write.vi"("requests"=w289, "OPC UA client refnum in"=w296) -> ()  [unwired: 6 in, 4 out]
          }
          event "ACTIVATE - CTAH": Value Change {
            w303 = T3 0 items=["Good"=0, "Uncertain_InitialValue"=1083310080, "Uncertain_LastUsableValue"=1083179008, "Uncertain_SensorNotAccurate"=1083375616, "Uncertain_EngineeringUnitsExceeded"=1083441152, "Bad_NoCommunication"=2150694912, "Bad_NotReadable"=2151284736, "Bad_NotWritable"=2151350272, "Bad_OutOfRange"=2151415808, "Bad_WaitingForInitialData"=2150760448] ("node status")
            n101 = event-data() -> ()  [unwired: 1 in, 6 out]
            n102 = Bundle By Name(cluster=T4 {"node ID"="", "value"=FALSE, "timestamp (current time)"=timestamp(0 s since 1904-01-01), "node status"=0} ("request"), "node ID"="s=activateCtah", "value"="ACTIVATE - CTAH", "timestamp (current time)"=timestamp(0 s since 1904-01-01), "node status"=w303) -> (w300:T4)
            n103 = Build Array(w300) -> (w299:T11)
            n104 = call-poly <vilib>:"Multiple Write.vi"("requests"=w299, "OPC UA client refnum in"=w297) -> ()  [unwired: 6 in, 4 out]
          }
          event "ACTIVATE - PUMP": Value Change {
            w311 = T3 0 items=["Good"=0, "Uncertain_InitialValue"=1083310080, "Uncertain_LastUsableValue"=1083179008, "Uncertain_SensorNotAccurate"=1083375616, "Uncertain_EngineeringUnitsExceeded"=1083441152, "Bad_NoCommunication"=2150694912, "Bad_NotReadable"=2151284736, "Bad_NotWritable"=2151350272, "Bad_OutOfRange"=2151415808, "Bad_WaitingForInitialData"=2150760448] ("node status")
            n105 = event-data() -> ()  [unwired: 1 in, 6 out]
            n106 = Bundle By Name(cluster=T4 {"node ID"="", "value"=FALSE, "timestamp (current time)"=timestamp(0 s since 1904-01-01), "node status"=0} ("request"), "node ID"="s=activatePump", "value"="ACTIVATE - PUMP", "timestamp (current time)"=timestamp(0 s since 1904-01-01), "node status"=w311) -> (w308:T4)
            n107 = Build Array(w308) -> (w307:T11)
            n108 = call-poly <vilib>:"Multiple Write.vi"("requests"=w307, "OPC UA client refnum in"=w305) -> ()  [unwired: 6 in, 4 out]
          }
          event "Pump Frequency [Hz]": Value Change {
            w320 = T3 0 items=["Good"=0, "Uncertain_InitialValue"=1083310080, "Uncertain_LastUsableValue"=1083179008, "Uncertain_SensorNotAccurate"=1083375616, "Uncertain_EngineeringUnitsExceeded"=1083441152, "Bad_NoCommunication"=2150694912, "Bad_NotReadable"=2151284736, "Bad_NotWritable"=2151350272, "Bad_OutOfRange"=2151415808, "Bad_WaitingForInitialData"=2150760448] ("node status")
            n109 = event-data() -> ()  [unwired: 1 in, 6 out]
            n110 = Bundle By Name(cluster=T5 {"node ID"="", "value"=0.0, "timestamp (current time)"=timestamp(0 s since 1904-01-01), "node status"=0} ("request"), "node ID"="s=pumpFrequency", "value"="Pump Frequency [Hz]", "timestamp (current time)"=timestamp(0 s since 1904-01-01), "node status"=w320) -> (w315:T5)
            n111 = Build Array(w315) -> (w313:T12)
            n112 = call-poly <vilib>:"Multiple Write.vi"("requests"=w313, "OPC UA client refnum in"=w317) -> ()  [unwired: 6 in, 4 out]
          }
          event "Desired Power [W]": Value Change {
            w323 = T3 0 items=["Good"=0, "Uncertain_InitialValue"=1083310080, "Uncertain_LastUsableValue"=1083179008, "Uncertain_SensorNotAccurate"=1083375616, "Uncertain_EngineeringUnitsExceeded"=1083441152, "Bad_NoCommunication"=2150694912, "Bad_NotReadable"=2151284736, "Bad_NotWritable"=2151350272, "Bad_OutOfRange"=2151415808, "Bad_WaitingForInitialData"=2150760448] ("node status")
            n113 = event-data() -> ()  [unwired: 1 in, 6 out]
            n114 = Bundle By Name(cluster=T5 {"node ID"="", "value"=0.0, "timestamp (current time)"=timestamp(0 s since 1904-01-01), "node status"=0} ("request"), "node ID"="s=desiredPower", "value"="Desired Power [W]", "timestamp (current time)"=timestamp(0 s since 1904-01-01), "node status"=w323) -> (w327:T5)
            n115 = Build Array(w327) -> (w328:T12)
            n116 = call-poly <vilib>:"Multiple Write.vi"("requests"=w328, "OPC UA client refnum in"=w321) -> ()  [unwired: 6 in, 4 out]
          }
          event "CTAH Set Point": Value Change {
            w331 = T3 0 items=["Good"=0, "Uncertain_InitialValue"=1083310080, "Uncertain_LastUsableValue"=1083179008, "Uncertain_SensorNotAccurate"=1083375616, "Uncertain_EngineeringUnitsExceeded"=1083441152, "Bad_NoCommunication"=2150694912, "Bad_NotReadable"=2151284736, "Bad_NotWritable"=2151350272, "Bad_OutOfRange"=2151415808, "Bad_WaitingForInitialData"=2150760448] ("node status")
            n117 = event-data() -> ()  [unwired: 1 in, 6 out]
            n118 = Bundle By Name(cluster=T5 {"node ID"="", "value"=0.0, "timestamp (current time)"=timestamp(0 s since 1904-01-01), "node status"=0} ("request"), "node ID"="s=ctahSetPoint", "value"="CTAH Set Point", "timestamp (current time)"=timestamp(0 s since 1904-01-01), "node status"=w331) -> (w335:T5)
            n119 = Build Array(w335) -> (w336:T12)
            n120 = call-poly <vilib>:"Multiple Write.vi"("requests"=w336, "OPC UA client refnum in"=w329) -> ()  [unwired: 6 in, 4 out]
          }
          event "TCHX Frequency [Hz]": Value Change {
            w339 = T3 0 items=["Good"=0, "Uncertain_InitialValue"=1083310080, "Uncertain_LastUsableValue"=1083179008, "Uncertain_SensorNotAccurate"=1083375616, "Uncertain_EngineeringUnitsExceeded"=1083441152, "Bad_NoCommunication"=2150694912, "Bad_NotReadable"=2151284736, "Bad_NotWritable"=2151350272, "Bad_OutOfRange"=2151415808, "Bad_WaitingForInitialData"=2150760448] ("node status")
            n121 = event-data() -> ()  [unwired: 1 in, 6 out]
            n122 = Bundle By Name(cluster=T5 {"node ID"="", "value"=0.0, "timestamp (current time)"=timestamp(0 s since 1904-01-01), "node status"=0} ("request"), "node ID"="s=tchxFrequency", "value"="TCHX Frequency [Hz]", "timestamp (current time)"=timestamp(0 s since 1904-01-01), "node status"=w339) -> (w343:T5)
            n123 = Build Array(w343) -> (w344:T12)
            n124 = call-poly <vilib>:"Multiple Write.vi"("requests"=w344, "OPC UA client refnum in"=w337) -> ()  [unwired: 6 in, 4 out]
          }
          event "Power Output On": Value Change {
            w351 = T3 0 items=["Good"=0, "Uncertain_InitialValue"=1083310080, "Uncertain_LastUsableValue"=1083179008, "Uncertain_SensorNotAccurate"=1083375616, "Uncertain_EngineeringUnitsExceeded"=1083441152, "Bad_NoCommunication"=2150694912, "Bad_NotReadable"=2151284736, "Bad_NotWritable"=2151350272, "Bad_OutOfRange"=2151415808, "Bad_WaitingForInitialData"=2150760448] ("node status")
            n125 = event-data() -> ()  [unwired: 1 in, 6 out]
            n126 = Bundle By Name(cluster=T4 {"node ID"="", "value"=FALSE, "timestamp (current time)"=timestamp(0 s since 1904-01-01), "node status"=0} ("request"), "node ID"="s=powerOutputOn", "value"="Power Output On", "timestamp (current time)"=timestamp(0 s since 1904-01-01), "node status"=w351) -> (w348:T4)
            n127 = Build Array(w348) -> (w347:T11)
            n128 = call-poly <vilib>:"Multiple Write.vi"("requests"=w347, "OPC UA client refnum in"=w345) -> ()  [unwired: 6 in, 4 out]
          }
          event "Exit Profile": Value Change {
            w359 = T3 0 items=["Good"=0, "Uncertain_InitialValue"=1083310080, "Uncertain_LastUsableValue"=1083179008, "Uncertain_SensorNotAccurate"=1083375616, "Uncertain_EngineeringUnitsExceeded"=1083441152, "Bad_NoCommunication"=2150694912, "Bad_NotReadable"=2151284736, "Bad_NotWritable"=2151350272, "Bad_OutOfRange"=2151415808, "Bad_WaitingForInitialData"=2150760448] ("node status")
            n129 = event-data() -> ()  [unwired: 1 in, 6 out]
            n130 = Bundle By Name(cluster=T4 {"node ID"="", "value"=FALSE, "timestamp (current time)"=timestamp(0 s since 1904-01-01), "node status"=0} ("request"), "node ID"="s=exitProfile", "value"="Exit Profile", "timestamp (current time)"=timestamp(0 s since 1904-01-01), "node status"=w359) -> (w356:T4)
            n131 = Build Array(w356) -> (w355:T11)
            n132 = call-poly <vilib>:"Multiple Write.vi"("requests"=w355, "OPC UA client refnum in"=w353) -> ()  [unwired: 6 in, 4 out]
          }
          event "Flow Data?": Value Change {
            w367 = T3 0 items=["Good"=0, "Uncertain_InitialValue"=1083310080, "Uncertain_LastUsableValue"=1083179008, "Uncertain_SensorNotAccurate"=1083375616, "Uncertain_EngineeringUnitsExceeded"=1083441152, "Bad_NoCommunication"=2150694912, "Bad_NotReadable"=2151284736, "Bad_NotWritable"=2151350272, "Bad_OutOfRange"=2151415808, "Bad_WaitingForInitialData"=2150760448] ("node status")
            n133 = event-data() -> ()  [unwired: 1 in, 6 out]
            n134 = Bundle By Name(cluster=T4 {"node ID"="", "value"=FALSE, "timestamp (current time)"=timestamp(0 s since 1904-01-01), "node status"=0} ("request"), "node ID"="s=activatePump", "value"="Flow Data?", "timestamp (current time)"=timestamp(0 s since 1904-01-01), "node status"=w367) -> (w364:T4)
            n135 = Build Array(w364) -> (w363:T11)
            n136 = call-poly <vilib>:"Multiple Write.vi"("requests"=w363, "OPC UA client refnum in"=w361) -> ()  [unwired: 6 in, 4 out]
          }
          event "Connect to Server": Value Change {
            n137 = event-data() -> ()  [unwired: 1 in, 6 out]
          }
          event "Disconnect": Value Change {
            n138 = event-data() -> ()  [unwired: 1 in, 6 out]
          }
          event "Stop": Value Change {
            n139 = event-data() -> ()  [unwired: 1 in, 6 out]
          }
        }
      }
      frame "Initialize" {
        w376 = FALSE  # Connection Status
        w377 = string[] []  # OPC UA Monitored Nodes
        w378 = T13 0  # OPC UA Subscription ID
        w379 = T10 0 items=["Good"=0, "Good_SubscriptionTransferred"=2949120, "Good_CompletesAsynchronously"=3014656, "Good_Overload"=3080192, "Good_Clamped"=3145728, "Good_LocalOverride"=9830400, "Good_EntryInserted"=10616832, "Good_EntryReplaced"=10682368, "Good_NoData"=10813440, "Good_MoreData"=10878976, "Good_CommunicationEvent"=10944512, "Good_ShutdownEvent"=11010048, "Good_CallAgain"=11075584, "Good_NonCriticalTimeout"=11141120, "Good_ResultsMayBeIncomplete"=12189696, "Good_DataIgnored"=14221312, "Uncertain"=1073741824, "Uncertain_ReferenceOutOfServer"=1080819712, "Uncertain_NoCommunicationLastUsableValue"=1083113472, "Uncertain_LastUsableValue"=1083179008, "Uncertain_SubstituteValue"=1083244544, "Uncertain_InitialValue"=1083310080, "Uncertain_SensorNotAccurate"=1083375616, "Uncertain_EngineeringUnitsExceeded"=1083441152, "Uncertain_SubNormal"=1083506688, "Uncertain_DataSubNormal"=1084489728, "Uncertain_ReferenceNotDeleted"=1086062592, "Uncertain_NotAllNodesAvailable"=1086324736, "Bad"=2147483648, "Bad_UnexpectedError"=2147549184, "Bad_InternalError"=2147614720, "Bad_OutOfMemory"=2147680256, "Bad_ResourceUnavailable"=2147745792, "Bad_CommunicationError"=2147811328, "Bad_EncodingError"=2147876864, "Bad_DecodingError"=2147942400, "Bad_EncodingLimitsExceeded"=2148007936, "Bad_UnknownResponse"=2148073472, "Bad_Timeout"=2148139008, "Bad_ServiceUnsupported"=2148204544, "Bad_Shutdown"=2148270080, "Bad_ServerNotConnected"=2148335616, "Bad_ServerHalted"=2148401152, "Bad_NothingToDo"=2148466688, "Bad_TooManyOperations"=2148532224, "Bad_DataTypeIdUnknown"=2148597760, "Bad_CertificateInvalid"=2148663296, "Bad_SecurityChecksFailed"=2148728832, "Bad_CertificateTimeInvalid"=2148794368, "Bad_CertificateIssuerTimeInvalid"=2148859904, "Bad_CertificateHostNameInvalid"=2148925440, "Bad_CertificateUriInvalid"=2148990976, "Bad_CertificateUseNotAllowed"=2149056512, "Bad_CertificateIssuerUseNotAllowed"=2149122048, "Bad_CertificateUntrusted"=2149187584, "Bad_CertificateRevocationUnknown"=2149253120, "Bad_CertificateIssuerRevocationUnknown"=2149318656, "Bad_CertificateRevoked"=2149384192, "Bad_CertificateIssuerRevoked"=2149449728, "Bad_UserAccessDenied"=2149515264, "Bad_IdentityTokenInvalid"=2149580800, "Bad_IdentityTokenRejected"=2149646336, "Bad_SecureChannelIdInvalid"=2149711872, "Bad_InvalidTimestamp"=2149777408, "Bad_NonceInvalid"=2149842944, "Bad_SessionIdInvalid"=2149908480, "Bad_SessionClosed"=2149974016, "Bad_SessionNotActivated"=2150039552, "Bad_SubscriptionIdInvalid"=2150105088, "Bad_RequestHeaderInvalid"=2150236160, "Bad_TimestampsToReturnInvalid"=2150301696, "Bad_RequestCancelledByClient"=2150367232, "Bad_NoCommunication"=2150694912, "Bad_WaitingForInitialData"=2150760448, "Bad_NodeIdInvalid"=2150825984, "Bad_NodeIdUnknown"=2150891520, "Bad_AttributeIdInvalid"=2150957056, "Bad_IndexRangeInvalid"=2151022592, "Bad_IndexRangeNoData"=2151088128, "Bad_DataEncodingInvalid"=2151153664, "Bad_DataEncodingUnsupported"=2151219200, "Bad_NotReadable"=2151284736, "Bad_NotWritable"=2151350272, "Bad_OutOfRange"=2151415808, "Bad_NotSupported"=2151481344, "Bad_NotFound"=2151546880, "Bad_ObjectDeleted"=2151612416, "Bad_NotImplemented"=2151677952, "Bad_MonitoringModeInvalid"=2151743488, "Bad_MonitoredItemIdInvalid"=2151809024, "Bad_MonitoredItemFilterInvalid"=2151874560, "Bad_MonitoredItemFilterUnsupported"=2151940096, "Bad_FilterNotAllowed"=2152005632, "Bad_StructureMissing"=2152071168, "Bad_EventFilterInvalid"=2152136704, "Bad_ContentFilterInvalid"=2152202240, "Bad_FilterOperandInvalid"=2152267776, "Bad_ContinuationPointInvalid"=2152333312, "Bad_NoContinuationPoints"=2152398848, "Bad_ReferenceTypeIdInvalid"=2152464384, "Bad_BrowseDirectionInvalid"=2152529920, "Bad_NodeNotInView"=2152595456, "Bad_ServerUriInvalid"=2152660992, "Bad_ServerNameMissing"=2152726528, "Bad_DiscoveryUrlMissing"=2152792064, "Bad_SempahoreFileMissing"=2152857600, "Bad_RequestTypeInvalid"=2152923136, "Bad_SecurityModeRejected"=2152988672, "Bad_SecurityPolicyRejected"=2153054208, "Bad_TooManySessions"=2153119744, "Bad_UserSignatureInvalid"=2153185280, "Bad_ApplicationSignatureInvalid"=2153250816, "Bad_NoValidCertificates"=2153316352, "Bad_RequestCancelledByRequest"=2153381888, "Bad_ParentNodeIdInvalid"=2153447424, "Bad_ReferenceNotAllowed"=2153512960, "Bad_NodeIdRejected"=2153578496, "Bad_NodeIdExists"=2153644032, "Bad_NodeClassInvalid"=2153709568, "Bad_BrowseNameInvalid"=2153775104, "Bad_BrowseNameDuplicated"=2153840640, "Bad_NodeAttributesInvalid"=2153906176, "Bad_TypeDefinitionInvalid"=2153971712, "Bad_SourceNodeIdInvalid"=2154037248, "Bad_TargetNodeIdInvalid"=2154102784, "Bad_DuplicateReferenceNotAllowed"=2154168320, "Bad_InvalidSelfReference"=2154233856, "Bad_ReferenceLocalOnly"=2154299392, "Bad_NoDeleteRights"=2154364928, "Bad_ServerIndexInvalid"=2154430464, "Bad_ViewIdUnknown"=2154496000, "Bad_TooManyMatches"=2154627072, "Bad_QueryTooComplex"=2154692608, "Bad_NoMatch"=2154758144, "Bad_MaxAgeInvalid"=2154823680, "Bad_HistoryOperationInvalid"=2154889216, "Bad_HistoryOperationUnsupported"=2154954752, "Bad_WriteNotSupported"=2155020288, "Bad_TypeMismatch"=2155085824, "Bad_MethodInvalid"=2155151360, "Bad_ArgumentsMissing"=2155216896, "Bad_TooManySubscriptions"=2155282432, "Bad_TooManyPublishRequests"=2155347968, "Bad_NoSubscription"=2155413504, "Bad_SequenceNumberUnknown"=2155479040, "Bad_MessageNotAvailable"=2155544576, "Bad_InsufficientClientProfile"=2155610112, "Bad_TcpServerTooBusy"=2155675648, "Bad_TcpMessageTypeInvalid"=2155741184, "Bad_TcpSecureChannelUnknown"=2155806720, "Bad_TcpMessageTooLarge"=2155872256, "Bad_TcpNotEnoughResources"=2155937792, "Bad_TcpInternalError"=2156003328, "Bad_TcpEndpointUrlInvalid"=2156068864, "Bad_RequestInterrupted"=2156134400, "Bad_RequestTimeout"=2156199936, "Bad_SecureChannelClosed"=2156265472, "Bad_SecureChannelTokenUnknown"=2156331008, "Bad_SequenceNumberInvalid"=2156396544, "Bad_ConfigurationError"=2156462080, "Bad_NotConnected"=2156527616, "Bad_DeviceFailure"=2156593152, "Bad_SensorFailure"=2156658688, "Bad_OutOfService"=2156724224, "Bad_DeadbandFilterInvalid"=2156789760, "Bad_RefreshInProgress"=2157379584, "Bad_ConditionAlreadyDisabled"=2157445120, "Bad_ConditionDisabled"=2157510656, "Bad_EventIdUnknown"=2157576192, "Bad_NoData"=2157641728, "Bad_DataLost"=2157772800, "Bad_DataUnavailable"=2157838336, "Bad_EntryExists"=2157903872, "Bad_NoEntryExists"=2157969408, "Bad_TimestampNotSupported"=2158034944, "Bad_InvalidArgument"=2158690304, "Bad_ConnectionRejected"=2158755840, "Bad_Disconnect"=2158821376, "Bad_ConnectionClosed"=2158886912, "Bad_InvalidState"=2158952448, "Bad_EndOfStream"=2159017984, "Bad_NoDataAvailable"=2159083520, "Bad_WaitingForResponse"=2159149056, "Bad_OperationAbandoned"=2159214592, "Bad_ExpectedStreamToBlock"=2159280128, "Bad_WouldBlock"=2159345664, "Bad_SyntaxError"=2159411200, "Bad_MaxConnectionsReached"=2159476736, "Bad_RequestTooLarge"=2159542272, "Bad_ResponseTooLarge"=2159607808, "Bad_EventNotAcknowledgeable"=2159738880, "Bad_InvalidTimestampArgument"=2159869952, "Bad_ProtocolVersionUnsupported"=2159935488, "Bad_StateNotActive"=2160001024, "Bad_FilterOperatorInvalid"=2160132096, "Bad_FilterOperatorUnsupported"=2160197632, "Bad_FilterOperandCountMismatch"=2160263168, "Bad_FilterElementInvalid"=2160328704, "Bad_FilterLiteralInvalid"=2160394240, "Bad_IdentityChangeNotSupported"=2160459776, "Bad_NotTypeDefinition"=2160590848, "Bad_ViewTimestampInvalid"=2160656384, "Bad_ViewParameterMismatch"=2160721920, "Bad_ViewVersionInvalid"=2160787456, "Bad_ConditionAlreadyEnabled"=2160852992, "Bad_DialogNotActive"=2160918528, "Bad_DialogResponseInvalid"=2160984064, "Bad_ConditionBranchAlreadyAcked"=2161049600, "Bad_ConditionBranchAlreadyConfirmed"=2161115136, "Bad_ConditionAlreadyShelved"=2161180672, "Bad_ConditionNotShelved"=2161246208, "Bad_ShelvingTimeOutOfRange"=2161311744, "Bad_AggregateListMismatch"=2161377280, "Bad_AggregateNotSupported"=2161442816, "Bad_AggregateInvalidInputs"=2161508352, "Bad_BoundNotFound"=2161573888, "Bad_BoundNotSupported"=2161639424, "Bad_AggregateConfigurationRejected"=2161770496, "Bad_TooManyMonitoredItems"=2161836032]  # OPC UA Subscription Service Status
        w380 = T7 refnum  # OPC UA client refnum
        w381 = refnum<event-registration> refnum  # OPC UA Data Change Event Registration Refnum
        n140 = Bundle(cluster=w374, "OPC UA Data Change Event Registration Refnum"=w381, "OPC UA client refnum"=w380, "OPC UA Subscription Service Status"=w379, "OPC UA Subscription ID"=w378, "OPC UA Monitored Nodes"=w377, "Connection Status"=w376) -> (w375:T14)
      }
      frame "Connect" {
        w383 = T15 ["s=Temperature", "s=Message", "s=Button", "s=fm40", "s=fm30", "s=wt20", "s=fm20", "s=fm60", "s=activateCtah", "s=desiredPower", "s=bt11", "s=st10", "s=cx101", "s=at01", "s=CTAHResGen", "s=ctahTempInResGen", "s=dhxTempOutResGen", "s=faultDiagnosticsActive", "s=heaterResGen", "s=heaterTempOutResGen", "s=outputCurrent1", "s=outputCurrent2", "s=outputVoltage1", "s=ouputVoltage2", "s=powerInputSignal", "s=powerOutput", "s=powerOutputOn", "s=actionRecorderOn", "s=exitProfile", "s=flowData", "s=spoofEnabled", "s=time", "s=chat", "s=operatorActions", "s=bt41", "i=20001", "s=bt12", "s=bt21", "s=bt23", "s=bt25", "s=bt27", "s=bt29", "s=bt30", "s=bt32", "s=bt34", "s=bt43", "s=bt60", "s=bt63", "s=bt65", "s=bt66", "s=cx102", "s=cx103", "s=cx104", "s=cx111", "s=cx112", "s=cx113", "s=cx114", "s=st11", "s=st12n", "s=st12se", "s=st12sw", "s=st13", "s=st14e", "s=st14n", "s=st14s", "s=st14w", "s=wt13", "s=wt20", "s=wt22", "s=wt24", "s=wt26", "s=wt28", "s=wt31", "s=wt33", "s=wt35", "s=wt40", "s=wt42", "s=wt61", "s=wt62", "s=wt64", "s=wt67", "s=activatePump", "s=activateTchx", "s=ctahFrequency", "s=ctahOperatingCase", "s=pumpFrequency", "s=pumpOperatingCase", "s=selectOperationMode", "s=tchxFrequency", "s=tchxOperatingCase", "s=at02", "s-desiredPower", "s=tchxFrequency", "s=ctahSetPoint"] ("node IDs")
        n141 = call <vilib>:"Connect.vi"("trust any server (F)"=TRUE, "error in (no error)"=w391, "security policy"=T6 {"message mode"=enum."None", "security"=enum."Basic256"}, "server endpoint URL"="opc.tcp://52.11.206.32:4840") -> ("error out"=w398:errorcluster, "OPC UA client refnum out"=w394:T7)  [unwired: 5 in, 1 out]
        n142 = call <vilib>:"Create Subscription.vi"("error in (no error)"=w398, "publishing interval (1000 ms)"=10.0, "OPC UA client refnum in"=w394) -> ("error out"=w399:errorcluster, "OPC UA data change event"=w401:refnum<user-event>, "subscription ID out"=w395:T13, "OPC UA client refnum out"=w400:T7)  [unwired: 4 in, 1 out]
        n143 = call <vilib>:"Add Monitored Data Nodes.vi"("error in (no error)"=w399, "node IDs"=w383, "subscription ID in"=w395, "OPC UA client refnum in"=w400) -> ("error out"=w385:errorcluster, "OPC UA client refnum out"=w396:T7)  [unwired: 4 in, 2 out]
        n144 = register-events(w401) -> (reference out=w397:refnum<event-registration>)  [unwired: 2 in, 1 out]
        n145 = Bundle By Name(cluster=w387, "OPC UA Monitored Nodes"=w383, "OPC UA Data Change Event Registration Refnum"=w397, "OPC UA client refnum"=w396, "OPC UA Subscription ID"=w395, "Connection Status"=TRUE) -> (w384:T14)
      }
      frame "Stop Check" {
        n146 = Unbundle By Name(w404) -> ("Connection Status"=w403:bool)
        n147 = case shown="True" w403 {
          tunnel: ["Stop" w411] -> w406
          frame False {
          }
          frame True {
            n148 = Two Button Dialog(message="The Server is still connected. You will need to disconnect before stopping. Would you like to disconnect?", 1:"No" ("F button name (\"Cancel\")"), 2:"Yes" ("T button name (\"OK\")")) -> (T button?=w409:bool)
            n149 = case shown="True" w409 {
              tunnel: ["Standby" "Disconnect and Stop"] -> w411
              frame False {
              }
              frame True {
              }
            }
          }
        }
      }
      frame "Disconnect" {
        n150 = Unbundle By Name(w418) -> ("OPC UA Monitored Nodes"=w430:string[], "OPC UA client refnum"=w429:T7, "OPC UA Subscription ID"=w428:T13)
        n151 = Bundle By Name(cluster=w418, "Connection Status"=FALSE) -> (w417:T14)
        n152 = call <vilib>:"Delete Monitored Nodes.vi"("error in (no error)"=w424, "node IDs"=w430, "subscription ID in"=w428, "OPC UA client refnum in"=w429) -> ("error out"=w423:errorcluster, "OPC UA client refnum out"=w426:T7)  [unwired: 3 in, 3 out]
        n153 = Build Array(w428) -> (w427:T13[])
        n154 = call <vilib>:"Delete Subscriptions.vi"("error in (no error)"=w423, "subscription IDs"=w427, "OPC UA client refnum in"=w426) -> ("error out"=w422:errorcluster, "OPC UA client refnum out"=w425:T7)  [unwired: 6 in, 1 out]
        n155 = call <vilib>:"Disconnect.vi"("error in (no error)"=w422, "OPC UA client refnum in"=w425) -> ("error out"=w419:errorcluster)  [unwired: 9 in]
      }
      frame "Disconnect and Stop" {
        n156 = Unbundle By Name(w433) -> ("OPC UA Monitored Nodes"=w445:string[], "OPC UA client refnum"=w444:T7, "OPC UA Subscription ID"=w443:T13)
        n157 = Bundle By Name(cluster=w433, "Connection Status"=FALSE) -> (w432:T14)
        n158 = call <vilib>:"Delete Monitored Nodes.vi"("error in (no error)"=w439, "node IDs"=w445, "subscription ID in"=w443, "OPC UA client refnum in"=w444) -> ("error out"=w438:errorcluster, "OPC UA client refnum out"=w441:T7)  [unwired: 3 in, 3 out]
        n159 = Build Array(w443) -> (w442:T13[])
        n160 = call <vilib>:"Delete Subscriptions.vi"("error in (no error)"=w438, "subscription IDs"=w442, "OPC UA client refnum in"=w441) -> ("error out"=w437:errorcluster, "OPC UA client refnum out"=w440:T7)  [unwired: 6 in, 1 out]
        n161 = call <vilib>:"Disconnect.vi"("error in (no error)"=w437, "OPC UA client refnum in"=w440) -> ("error out"=w434:errorcluster)  [unwired: 9 in]
      }
      frame "Stop" {
      }
    }
    n162 = Or(x=w11, y=w9) -> (x .or. y?=w10:bool)
  }
  n163 = call <vilib>:"Simple Error Handler.vi"("error in (no error)"=w2) -> ()  [unwired: 4 in, 5 out]
